vi "Velocity Trapezoid Calculations.vi"(9 "Distance":dbl, 10 "Velocity Max":dbl, 11 "Acceleration Max":dbl) -> (2 "Velocity values":dbl[](array[numeric]), 3 "Timestamp":dbl[](array[numeric]) format="%.2f")   [LabVIEW 2023]
panel:
  out "Time":sgl
  out "XY Graph":cluster{dbl[], dbl[]}(graph)
  out "Time(othy) (in seconds)":dbl
  # "*timeothy is the point where the slope changes in a trapezoid"
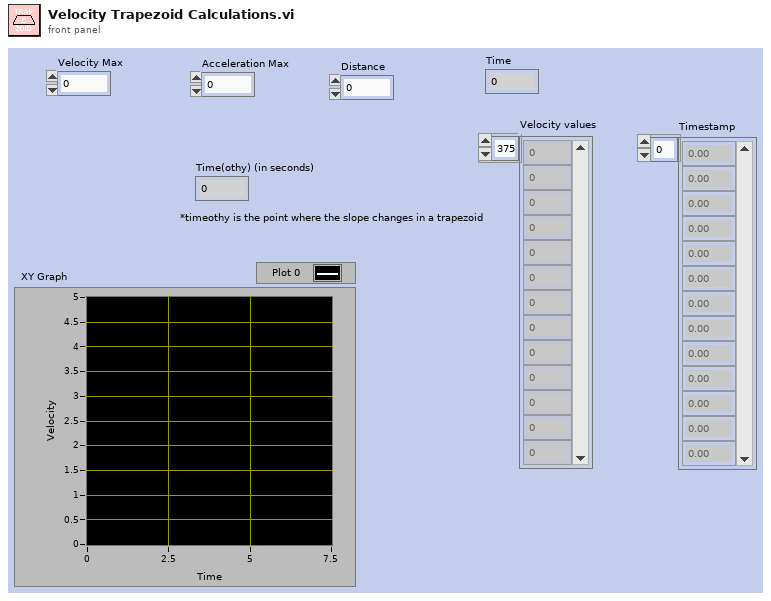
[diagram p1: front panel]
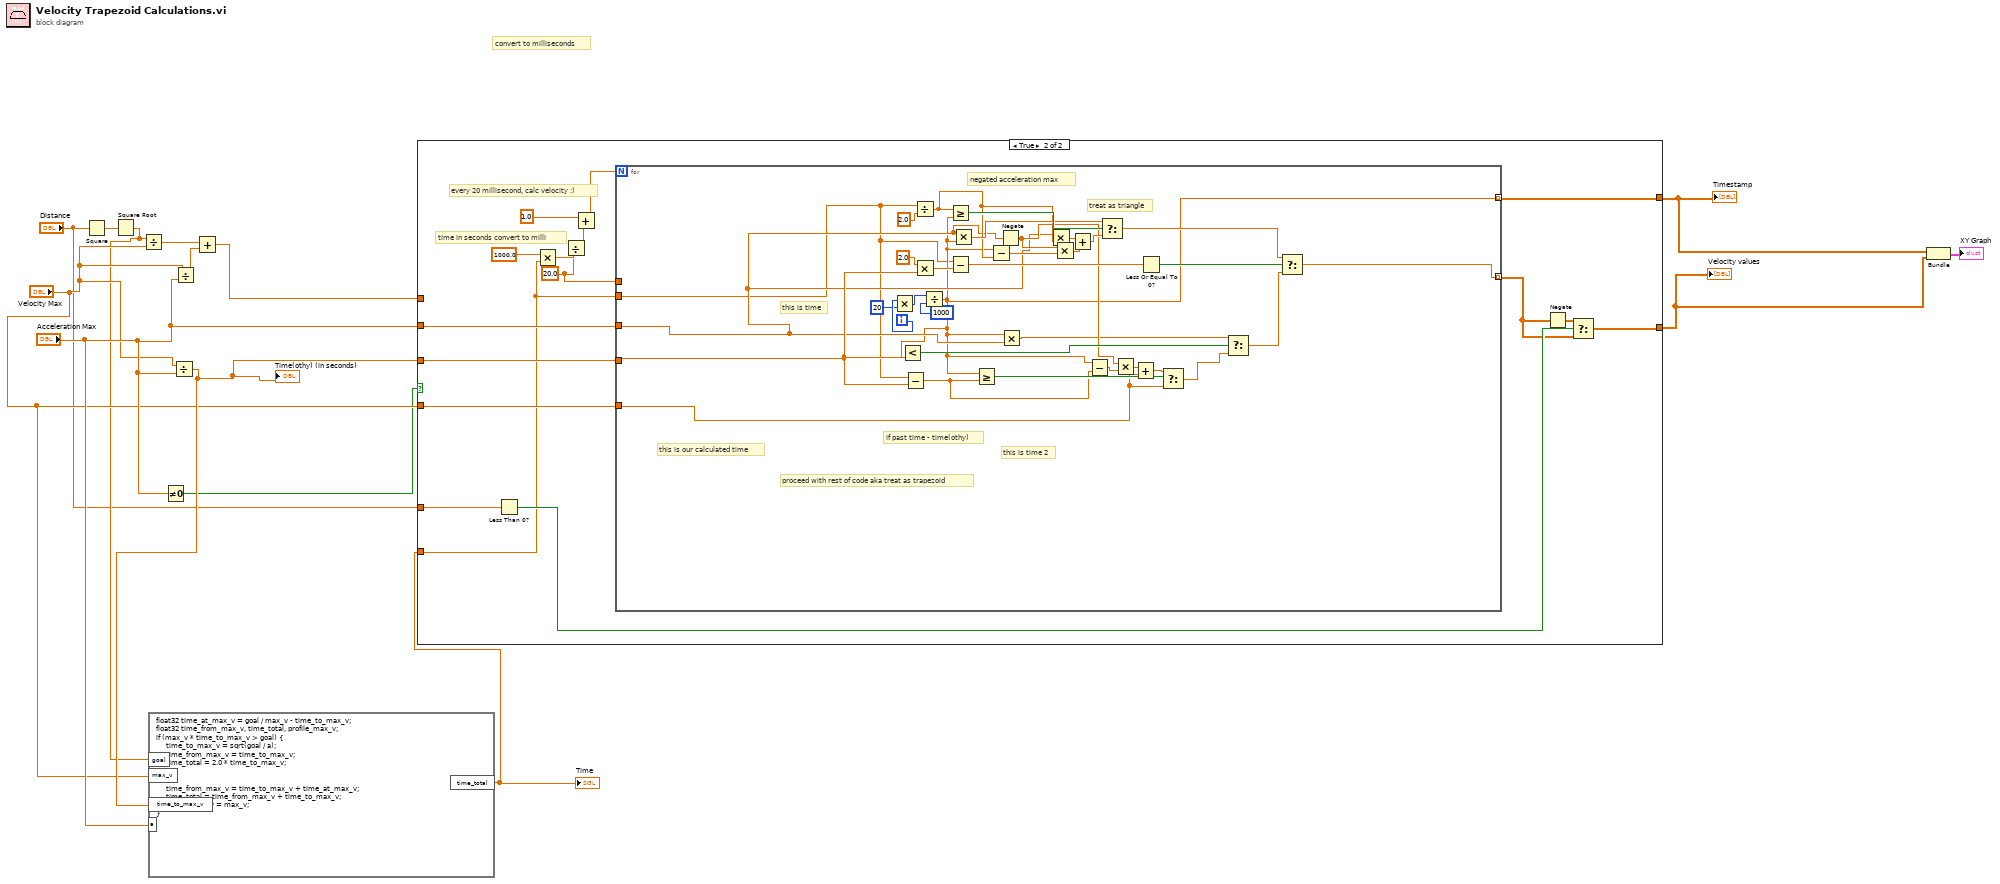
[diagram p0: block diagram]
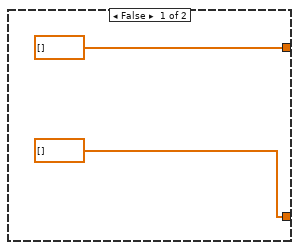
[diagram p2: hidden frame]
diagram:
  # "convert to milliseconds"
  n1 = Square(x="Distance") -> (x^2=w3:dbl)
  n2 = Square Root(x=w3) -> (sqrt(x)=w2:dbl)
  n3 = Divide(x=w2, y="Velocity Max") -> (x/y=w11:dbl)
  n4 = Not Equal To 0?(x="Acceleration Max") -> (x != 0?=w4:bool)
  n5 = Divide(x="Velocity Max", y="Acceleration Max") -> (x/y=w6:dbl)
  "Time(othy) (in seconds)" <- w6
  n6 = formula code="float32 time_at_max_v = goal / max_v - time_to_max_v;\nfloat32 time_from_max_v, time_total, profile_max_v;\nif (max_v * time_to_max_v > goal) {\n     time_to_max_v = sqrt(goal / a);\n     time_from_max_v = time_to_max_v;\n     time_total = 2.0 * time_to_max_v;\n}\nelse {\n     time_from_max_v = time_to_max_v + time_at_max_v;\n     time_total = time_from_max_v + time_to_max_v;\n     profile_max_v = max_v;\n}"("goal"=w2, "max_v"="Velocity Max", "time_to_max_v"=w6, "a"="Acceleration Max") -> ("time_total"=w8:sgl)
  "Time" <- w8
  n7 = Divide(x="Velocity Max", y="Acceleration Max") -> (x/y=w14:dbl)
  n8 = Add(x=w11, y=w14) -> (x+y=w12:dbl)
  n9 = case shown="True" w4 {
    tunnel: "Velocity Max" -> [_ w32]
    tunnel: w6 -> [_ w31]
    tunnel: [dbl[] [] w29] -> w13
    tunnel: w12 -> [_ _]
    tunnel: "Acceleration Max" -> [_ w25]
    tunnel: [dbl[] [] w21] -> w10
    tunnel: w8 -> [_ w18]
    tunnel: "Distance" -> [_ w19]
    frame False {
    }
    frame True {
      w20 = 20.0 ("y")
      # "every 20 millisecond, calc velocity :)"
      # "time in seconds convert to milli"
      n10 = Less Than 0?(x=w19) -> (x < 0?=w23:bool)
      n11 = Multiply(x=1000.0, y=w18) -> (x*y=w30:dbl)
      n12 = Divide(x=w30, y=w20) -> (x/y=w26:dbl)
      n13 = Add(x=1.0, y=w26) -> (x+y=w28:dbl)
      n14 = for {
        N: w28 -> [_]
        tunnel: [w55] -> w22 mode=indexing
        tunnel: w25 -> [w45]
        tunnel: w32 -> [w37]
        tunnel: w31 -> [w54]
        tunnel: [w35] -> w29 mode=indexing
        tunnel: w20 -> [_]
        tunnel: w18 -> [w34]
        i -> [w36]
        # "this is our calculated time"
        # "this is time 2"
        # "this is time"
        # "negated acceleration max"
        # "if past time - time(othy)"
        # "treat as triangle"
        # "proceed with rest of code aka treat as trapezoid"
        n15 = Multiply(x=w36, y=20) -> (x*y=w42:i32)
        n16 = Subtract(x=w34, y=w54) -> (x-y=w43:dbl)
        n17 = Divide(x=w34, y=2.0) -> (x/y=w48:dbl)
        n18 = Multiply(x=2.0, y=w54) -> (x*y=w64:dbl)
        n19 = Divide(x=w42, y=1000) -> (x/y=w35:dbl)
        n20 = Less?(x=w35, y=w54) -> (x < y?=w56:bool)
        n21 = Greater Or Equal?(x=w48, y=w35) -> (x >= y?=w60:bool)
        n22 = Subtract(x=w34, y=w64) -> (x-y=w63:dbl)
        n23 = Multiply(x=w45, y=w35) -> (x*y=w53:dbl)
        n24 = Greater Or Equal?(x=w35, y=w43) -> (x >= y?=w59:bool)
        n25 = Subtract(x=w35, y=w48) -> (x-y=w52:dbl)
        n26 = Negate(x=w45) -> (-x=w47:dbl)
        n27 = Multiply(x=w35, y=w45) -> (x*y=w40:dbl)
        n28 = Multiply(x=w45, y=w48) -> (x*y=w50:dbl)
        n29 = Multiply(x=w47, y=w52) -> (x*y=w51:dbl)
        n30 = Add(x=w50, y=w51) -> (x+y=w49:dbl)
        n31 = Subtract(x=w35, y=w43) -> (x-y=w38:dbl)
        n32 = Select(t=w53, s=w60, f=w49) -> (s? t:f=w44:dbl)
        n33 = Multiply(x=w47, y=w38) -> (x*y=w46:dbl)
        n34 = Add(x=w46, y=w37) -> (x+y=w39:dbl)
        n35 = Less Or Equal To 0?(x=w63) -> (x <= 0?=w62:bool)
        n36 = Select(t=w39, s=w59, f=w37) -> (s? t:f=w58:dbl)
        n37 = Select(t=w40, s=w56, f=w58) -> (s? t:f=w57:dbl)
        n38 = Select(t=w44, s=w62, f=w57) -> (s? t:f=w55:dbl)
      }
      n39 = Negate(x=w22) -> (-x=w24:dbl[])
      n40 = Select(t=w24, s=w23, f=w22) -> (s? t:f=w21:dbl[])
    }
  }
  "Velocity values" <- w10
  "Timestamp" <- w13
  n41 = Bundle(w13, w10) -> (→"XY Graph":cluster{dbl[], dbl[]})  [unwired: 1 in]
